vi "switchOn.vi"(8 "error in (no error)":errorcluster, 11 "Xcite in":refnum<class "Xcite.lvclass">) -> (0 "error out":errorcluster, 3 "Xcite out":refnum<class "Xcite.lvclass">)   [LabVIEW 2019, in "Xcite.lvclass"]
doc: "Switches on the XCite device output."
uses:
  Xcite.lvclass
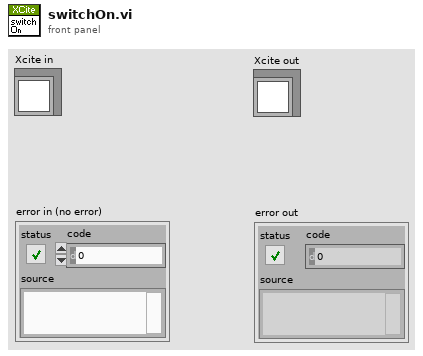
[diagram p1: front panel]
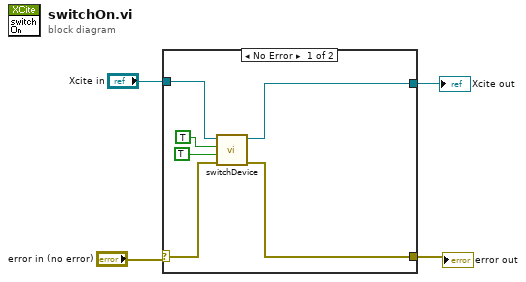
[diagram p0: block diagram]
diagram:
  n1 = case shown="No Error" "error in (no error)" {
    selector: "error in (no error)" -> [w10 w12]
    tunnel: [w9 w12] -> w3
    tunnel: "Xcite in" -> [w8 w11]
    tunnel: [w7 w11] -> w1
    frame No Error {
      n2 = call "switchDevice.vi"("error in (no error)"=w10, "on"=TRUE, "use_common_on_off"=TRUE, "Xcite in"=w8) -> ("error out"=w9:errorcluster, "Xcite out"=w7:refnum<class "Xcite.lvclass">)  [unwired: 6 in]
    }
    frame Error {
    }
  }
  "Xcite out" <- w1
  "error out" <- w3
